vi "Initialize.vi"(8 "error in (no error)":errorcluster, 11 "Game in":refnum<class "Game.lvclass">) -> (0 "error out":errorcluster, 3 "Game out":refnum<class "Game.lvclass">)   [LabVIEW 2015, in "TronviewGame.lvlib" / "Game.lvclass"]
uses:
  Game.lvclass
  Board/Position.ctl
  Game.lvclass/Game.ctl
  Board/GetBoardCenter.vi
  Board/Board.lvclass
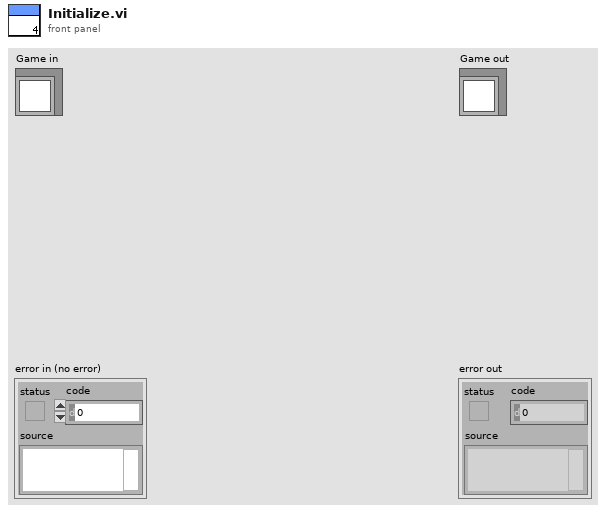
[diagram p1: front panel]
types:
  T1 = typedef "TronviewGame.lvlib/Board.lvclass/Position.ctl" = cluster{"Column":i32, "Row":i32}
  T2 = typedef "TronviewGame.lvlib/BotVIRefnum.ctl" = refnum<vi>
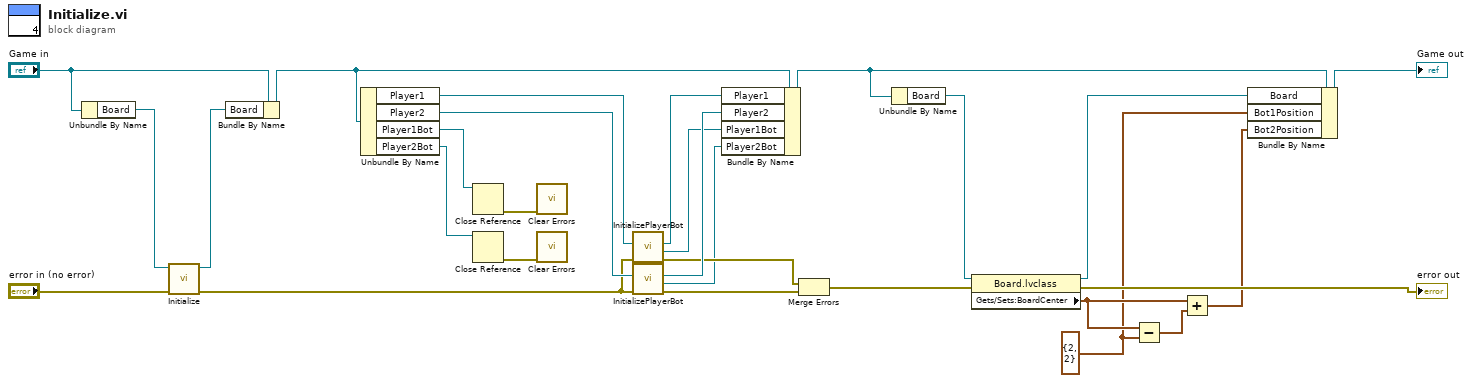
[diagram p0: block diagram]
diagram:
  w1 = T1 {"Column"=2, "Row"=2} ("Position")
  n1 = Unbundle By Name("Game in") -> ("Board"=w25:refnum<class "Board.lvclass">)
  n2 = call "Initialize.vi"("error in (no error)"="error in (no error)", "Board in"=w25) -> ("error out"=w14:errorcluster, "Board out"=w24:refnum<class "Board.lvclass">)  [unwired: 8 in]
  n3 = Bundle By Name(cluster="Game in", "Board"=w24) -> (w10:refnum<class "Game.lvclass">)
  n4 = Unbundle By Name(w10) -> ("Player1"=w23:refnum<class "Player.lvclass">, "Player2"=w22:refnum<class "Player.lvclass">, "Player1Bot"=w19:T2, "Player2Bot"=w18:T2)
  n5 = Close Reference(reference=w19) -> (error out=w17:errorcluster)  [unwired: 1 in]
  n6 = Close Reference(reference=w18) -> (error out=w16:errorcluster)  [unwired: 1 in]
  n7 = call <vilib>:"Clear Errors.vi"("error in (no error)"=w17) -> ()  [unwired: 5 in, 2 out]
  n8 = call <vilib>:"Clear Errors.vi"("error in (no error)"=w16) -> ()  [unwired: 5 in, 2 out]
  n9 = call "InitializePlayerBot.vi"("error in (no error)"=w14, "Player in"=w23) -> ("error out"=w15:errorcluster, "BotVIRefnum"=w11:T2, "Player out"=w20:refnum<class "Player.lvclass">)  [unwired: 7 in]
  n10 = call "InitializePlayerBot.vi"("error in (no error)"=w14, "Player in"=w22) -> ("error out"=w13:errorcluster, "BotVIRefnum"=w12:T2, "Player out"=w21:refnum<class "Player.lvclass">)  [unwired: 7 in]
  n11 = Bundle By Name(cluster=w10, "Player1"=w20, "Player2"=w21, "Player1Bot"=w11, "Player2Bot"=w12) -> (w9:refnum<class "Game.lvclass">)
  n12 = Merge Errors(w15, w13) -> (w27:errorcluster)
  n13 = Unbundle By Name(w9) -> ("Board"=w6:refnum<class "Board.lvclass">)
  n14 = property class="Board.lvclass"(reference=w6, error in=w27) -> (reference out=w5:refnum<class "Board.lvclass">, error out=→"error out":errorcluster, "Gets/Sets:BoardCenter"=w4:T1)
  n15 = Subtract(x=w4, y=w1) -> (x-y=w3:T1)
  n16 = Add(x=w4, y=w3) -> (x+y=w2:T1)
  n17 = Bundle By Name(cluster=w9, "Board"=w5, "Bot1Position"=w1, "Bot2Position"=w2) -> (→"Game out":refnum<class "Game.lvclass">)
